vi "ERASE Script-Completo.vi"(8 "error in (no error)":errorcluster, 11 "VISA resource name":refnum<visa-resource-name>) -> (0 "error out":errorcluster, 3 "VISA resource name out":refnum<visa-resource-name>)   [LabVIEW 2014, in "CAP-USB.lvlib"]
doc: "Envia el comando al CAP-USB\npara que borre el script que tiene cargado \nactualmente.\nAntes de poder borrar un script, se debe enviar el \ncomando STOP script"
uses:
  CAP-USB.lvlib
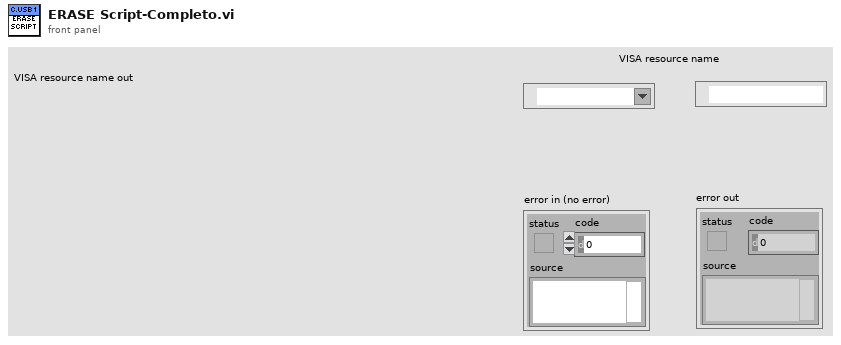
[diagram p1: front panel]
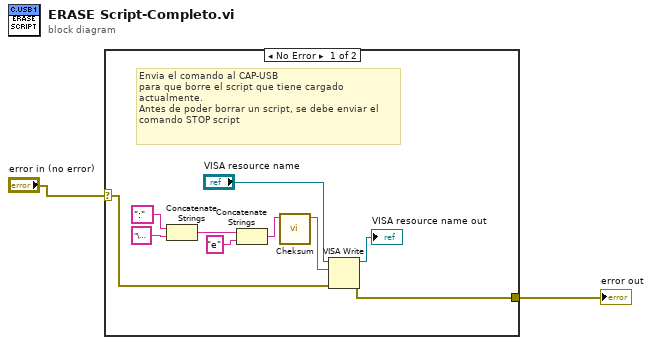
[diagram p0: block diagram]
diagram:
  n1 = case shown="No Error" "error in (no error)" {
    selector: "error in (no error)" -> [w3 w13]
    tunnel: [w10 w13] -> w2
    frame No Error {
      # "Envia el comando al CAP-USB\npara que borre el script que tiene cargado \nactualmente.\nAntes de poder borrar un script, se debe enviar el \ncomando STOP script"
      n2 = Concatenate Strings(":" ("COMANDO (e)"), "\u0001" ("COMANDO (e)")) -> (w7:string)
      n3 = Concatenate Strings(w7, "e" ("COMANDO (e)")) -> (w5:string)
      n4 = call "Cheksum.vi"("Trama IN"=w5) -> ("Trama RTS"=w4:string)  [unwired: 9 in, 1 out]
      n5 = VISA Write(VISA resource name="VISA resource name", write buffer=w4, error in (no error)=w3) -> (VISA resource name out=→"VISA resource name out":refnum<visa-resource-name>, error out=w10:errorcluster)  [unwired: 1 out]
    }
    frame Error {
    }
  }
  "error out" <- w2
